vi "myRIO v1.0 Open Writing DMA.vi"(8 "error in (no error)":errorcluster) -> (0 "error out":errorcluster)   [LabVIEW 2021]
uses:
  <vilib>/myRIO/Common/Instrument Driver Framework/Utilities/typedefs/Ref Counter Action Enum.ctl
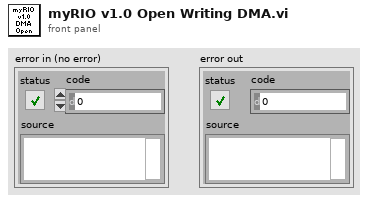
[diagram p1: front panel]
types:
  T1 = typedef "Ref Counter Action Enum.ctl" = enum16{"Set", "Get", "Increment", "Decrement"}
  T2 = typedef "Block Write Resource.ctl" = refnum<vi>
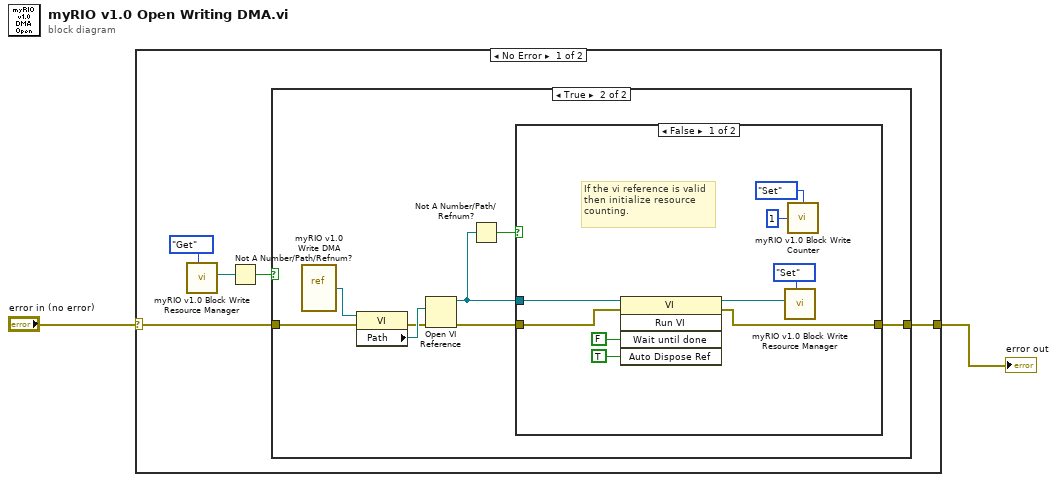
[diagram p0: block diagram]
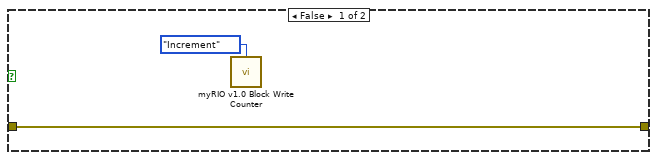
[diagram p2: hidden frame]
diagram:
  n1 = case shown="No Error" "error in (no error)" {
    selector: "error in (no error)" -> [w4 w28]
    tunnel: [w7 w28] -> w2
    frame No Error {
      n2 = call <vilib>:"myRIO v1.0 Block Write Resource Manager.vi"("Action"=enum16{"Get", "Set", "Reset"}."Get" ("Enum")) -> ("Resource Data Out"=w3:T2)  [unwired: 10 in]
      n3 = Not A Number/Path/Refnum?(number/path/refnum=w3) -> (NaN/Path/Refnum?=w5:bool)
      n4 = case shown="True" w5 {
        tunnel: [w9 w10] -> w7
        tunnel: w4 -> [w9 w14]
        frame False {
          n5 = call <vilib>:"myRIO v1.0 Block Write Counter.vi"("Resource Counter Action Enum"=Ref_Counter_Action_Enum."Increment") -> ()  [unwired: 1 in, 1 out]
        }
        frame True {
          n6 = vi-ref <vilib>:"myRIO v1.0 Write DMA.vi"() -> (w17:refnum<vi>)
          n7 = property class="VI"(reference=w17, error in=w14) -> (error out=w15:errorcluster, "Path"=w16:path)  [unwired: 1 out]
          n8 = Open VI Reference(vi path=w16, error in (no error)=w15) -> (vi reference=w12:refnum<vi>, error out=w11:errorcluster)  [unwired: 4 in]
          n9 = Not A Number/Path/Refnum?(number/path/refnum=w12) -> (NaN/Path/Refnum?=w13:bool)
          n10 = case shown="False" w13 {
            tunnel: w12 -> [w23 _]
            tunnel: w11 -> [w22 w27]
            tunnel: [w19 w27] -> w10
            frame False {
              # "If the vi reference is valid\nthen initialize resource\ncounting."
              n11 = invoke class="VI" method="Run VI"(reference=w23, error in=w22, "Wait until done"=FALSE ("Wait Until Done"), "Auto Dispose Ref"=TRUE ("Auto Dispose Reference")) -> (reference out=w18:refnum<vi>, error out=w19:errorcluster)  [unwired: 1 in, 3 out]
              n12 = call <vilib>:"myRIO v1.0 Block Write Resource Manager.vi"("Action"=enum16{"Get", "Set", "Reset"}."Set" ("Enum"), "Resource Data In"=w18) -> ()  [unwired: 9 in, 1 out]
              n13 = call <vilib>:"myRIO v1.0 Block Write Counter.vi"("Resource Count in"=u32 1, "Resource Counter Action Enum"=Ref_Counter_Action_Enum."Set") -> ()  [unwired: 1 out]
            }
            frame True {
              # "No error is thrown since the error will be generated by the Open node."
            }
          }
        }
      }
    }
    frame Error {
    }
  }
  "error out" <- w2
